vi "ConvertItemListToCalculateFormatElements.vi"(11 "Item List":string) -> (3 "Calculate Format Elements":T1[](array[typedef]))   [LabVIEW 2012, in "Keithley-6482.lvlib"]
uses:
  Public/Controls/CalculateFormatElement.ctl
  Keithley-6482.lvlib
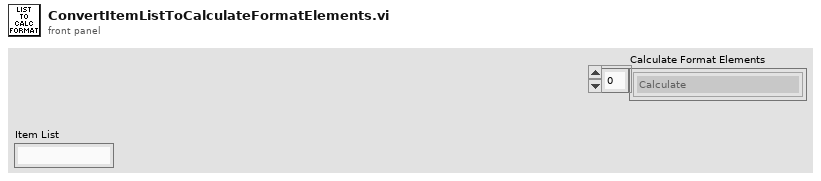
[diagram p1: front panel]
types:
  T1 = typedef "Keithley-6482.lvlib/CalculateFormatElement.ctl" = enum16{"Calculate", "Time", "Status"}
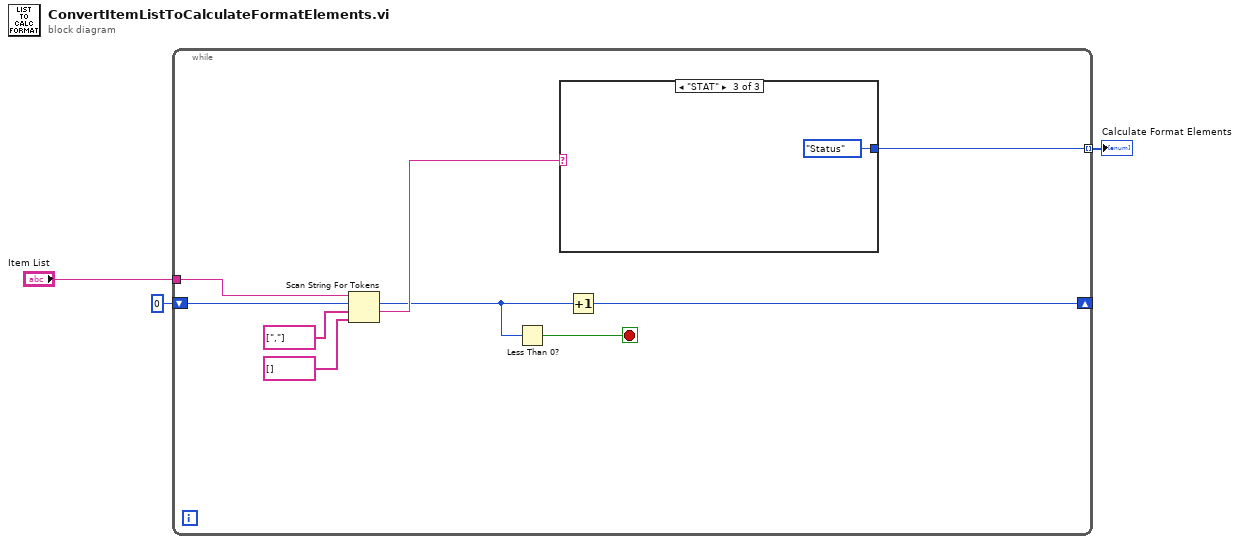
[diagram p0: block diagram]
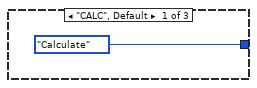
[diagram p2: hidden frame]
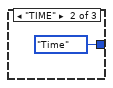
[diagram p3: hidden frame]
diagram:
  n1 = while {
    shift-right: [w5] -> _
    shift-left: 0 ("offset past token") -> [w12]
    tunnel: "Item List" -> [w8]
    tunnel: [w4] -> w1 mode=indexing
    stop <- w7 stop-if-true
    n2 = Scan String For Tokens(6:string[] [] ("delimiters (\\s,\\t,\\r,\\n)"), 7:string[] [","] ("delimiters (\\s,\\t,\\r,\\n)"), 8:w12, 9:w8) -> (1:w11:string, 2:w6:i32)  [unwired: 2 in, 2 out]
    n3 = Less Than 0?(x=w6) -> (x < 0?=w7:bool)
    n4 = case shown="\"STAT\"" w11 {
      tunnel: [CalculateFormatElement."Calculate" ("Calculate Format Element") CalculateFormatElement."Time" ("Calculate Format Element") CalculateFormatElement."Status" ("Calculate Format Element")] -> w4
      frame "CALC", Default {
      }
      frame "TIME" {
      }
      frame "STAT" {
      }
    }
    n5 = Increment(x=w6) -> (x+1=w5:i32)
  }
  "Calculate Format Elements" <- w1
